vi "ConfigMain_Dash.vi"(10 "ControlsToSave":refnum<vi>[](array[refnum]), 11 "ControlElements":T1) -> ()   [LabVIEW 2015]
uses:
  <vilib>/Rock Robotics/Network Tables/NT Write Boolean.vi
  <vilib>/FTP/NI_FTP.lvlib
panel:
  out "RobotIP":string
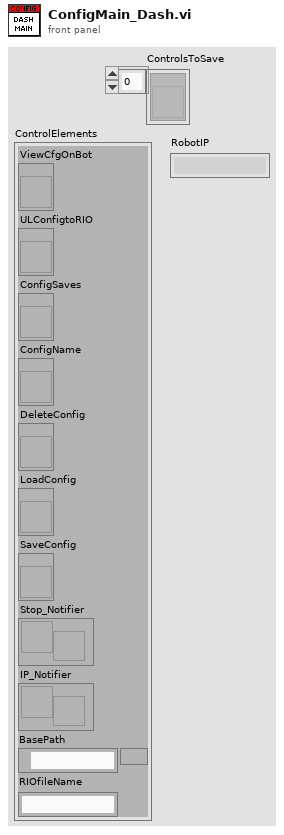
[diagram p1: front panel]
types:
  T1 = cluster{"ViewCfgOnBot":refnum<vi>, "ULConfigtoRIO":refnum<vi>, "ConfigSaves":refnum<vi>, "ConfigName":refnum<vi>, "DeleteConfig":refnum<vi>, "LoadConfig":refnum<vi>, "SaveConfig":refnum<vi>, "Stop_Notifier":refnum<notifier>, "IP_Notifier":refnum<notifier>, "BasePath":path, "RIOfileName":string}
  T2 = enum16{"open", "replace", "create", "open or create", "replace or create", "replace or create with confirmation"}
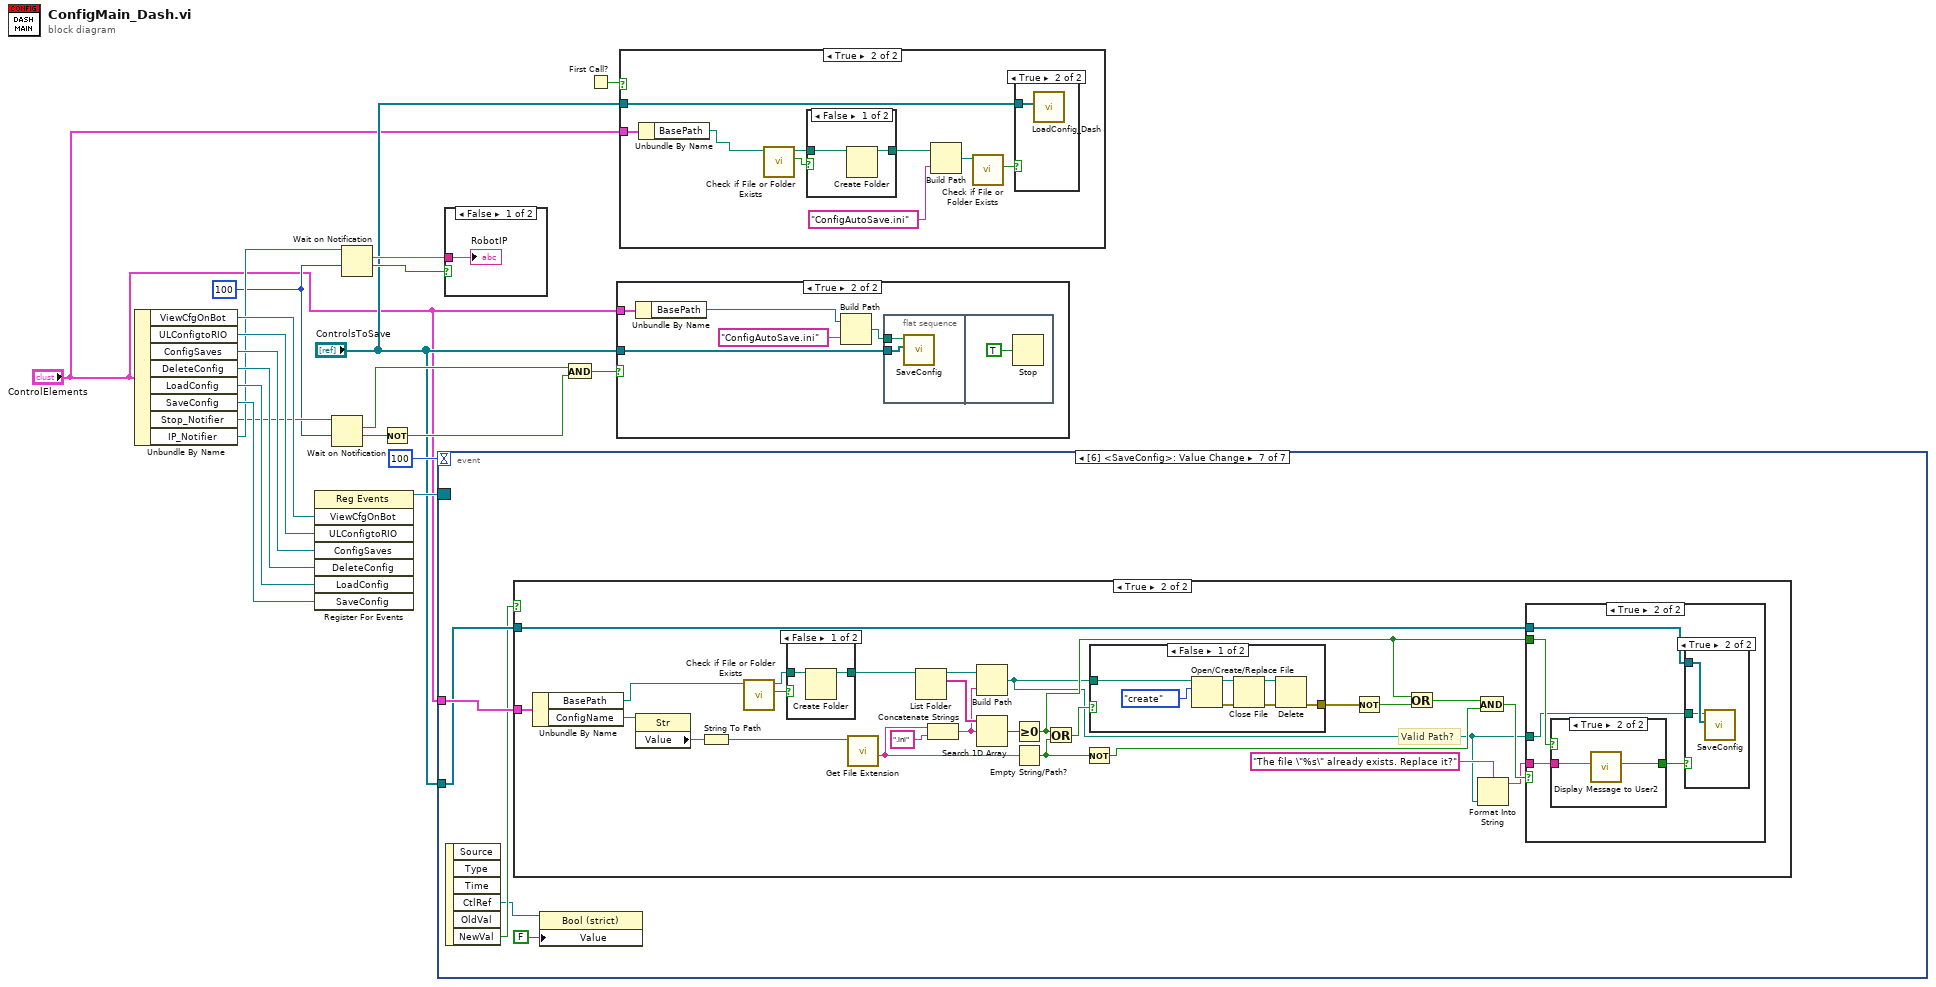
[diagram p0: block diagram]
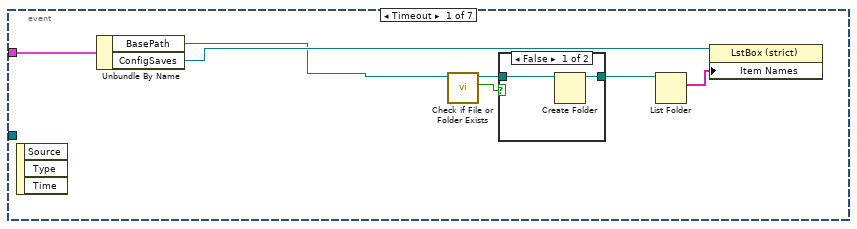
[diagram p7: hidden frame]
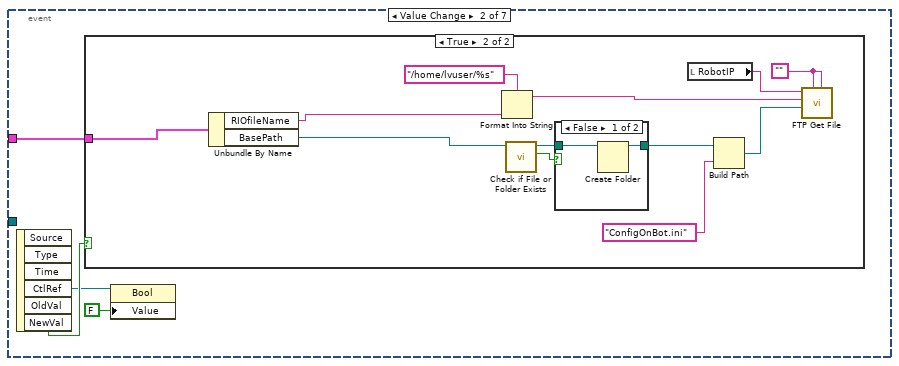
[diagram p9: hidden frame]
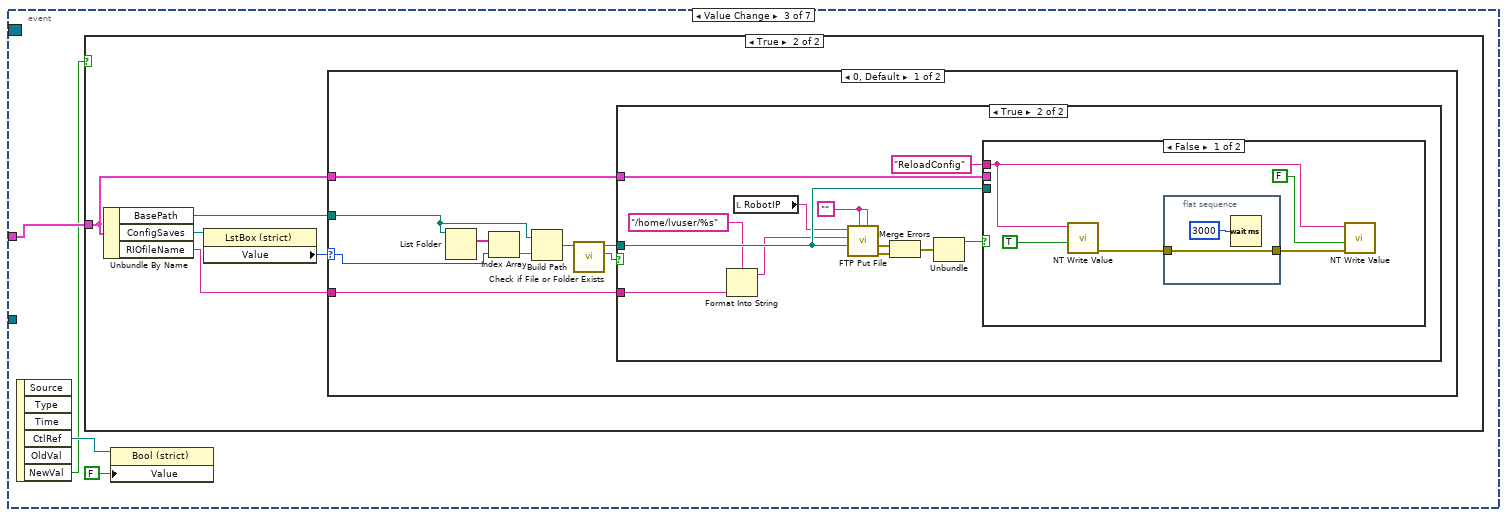
[diagram p12: hidden frame]
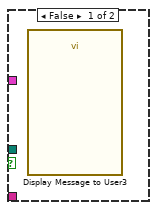
[diagram p14: hidden frame]
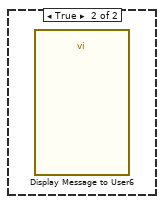
[diagram p15: hidden frame]
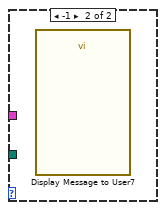
[diagram p16: hidden frame]
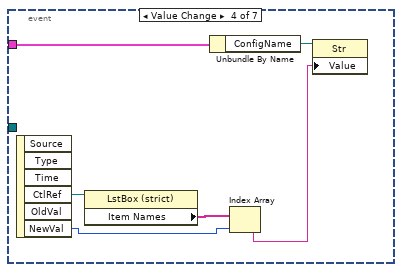
[diagram p17: hidden frame]
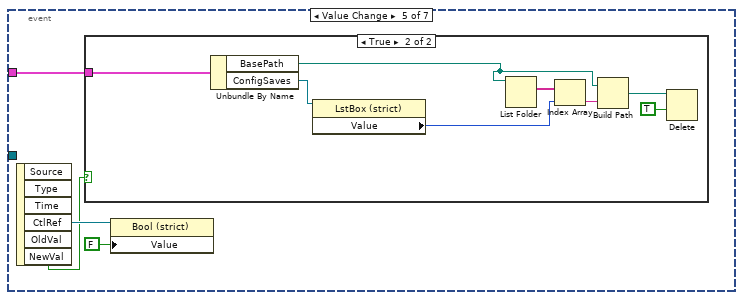
[diagram p18: hidden frame]
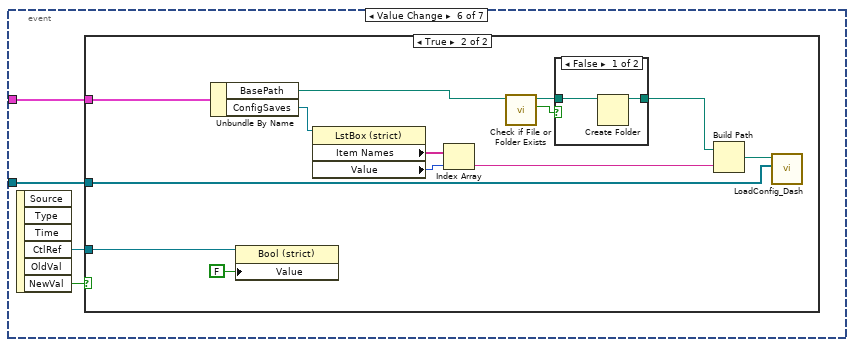
[diagram p20: hidden frame]
diagram:
  w9 = 100 ("timeout in ms (-1)")
  n1 = Unbundle By Name("ControlElements") -> ("ViewCfgOnBot"=w20:refnum<vi>, "ULConfigtoRIO"=w19:refnum<vi>, "ConfigSaves"=w18:refnum<vi>, "DeleteConfig"=w17:refnum<vi>, "LoadConfig"=w16:refnum<vi>, "SaveConfig"=w15:refnum<vi>, "Stop_Notifier"=w13:refnum<notifier>, "IP_Notifier"=w14:refnum<notifier>)
  n2 = register-events(w20, w19, w18, w17, w16, w15) -> (reference out=w12:refnum<event-registration>)  [unwired: 2 in, 1 out]
  n3 = Wait on Notification(notifier=w13, timeout in ms (-1)=w9) -> (notification=w6:bool, timed out?=w8:bool)  [unwired: 2 in, 2 out]
  n4 = Wait on Notification(notifier=w14, timeout in ms (-1)=w9) -> (notification=w11:string, timed out?=w10:bool)  [unwired: 2 in, 2 out]
  n5 = Not(x=w8) -> (.not. x?=w7:bool)
  n6 = event shown="[6] <SaveConfig>: Value Change" {
    selector: w12 -> [_ _ _ _ _ _ _]
    dyn-events: _ -> [_ _ _ _ _ _ _]
    timeout: 100 -> [_ _ _ _ _ _ _]
    tunnel: "ControlElements" -> [w26 w34 w52 w87 w93 w106 w129]
    tunnel: "ControlsToSave" -> [_ _ _ _ _ w105 w128]
    event Timeout {
      n7 = event-data() -> ()  [unwired: 1 in, 3 out]
      n8 = Unbundle By Name(w26) -> ("BasePath"=w21:path, "ConfigSaves"=w27:refnum<vi>)
      n9 = call <vilib>:"Check if File or Folder Exists.vi"("path"=w21) -> ("file or folder exists?"=w24:bool, "dup path"=w23:path)  [unwired: 8 in, 1 out]
      n10 = case shown="False" w24 {
        tunnel: w23 -> [w29 w30]
        tunnel: [w28 w30] -> w22
        frame False {
          n11 = Create Folder(path (use dialog)=w29) -> (created path=w28:path)  [unwired: 2 in, 2 out]
        }
        frame True {
        }
      }
      n12 = List Folder(path=w22) -> (filenames=w25:string[])  [unwired: 3 in, 3 out]
      n13 = property class="LstBox (strict)"(reference=w27, "Item Names"=w25) -> ()  [unwired: 1 in, 2 out]
    }
    event Value Change {
      n14 = event-data() -> ("CtlRef"=w31:refnum<vi>, "NewVal"=w33:bool)  [unwired: 1 in, 4 out]
      n15 = case shown="True" w33 {
        tunnel: w34 -> [_ w40]
        frame False {
        }
        frame True {
          w44 = ""
          n16 = Unbundle By Name(w40) -> ("RIOfileName"=w37:string, "BasePath"=w35:path)
          n17 = Format Into String(format string="/home/lvuser/%s" ("remote path"), w37) -> (resulting string=w36:string)  [unwired: 2 in, 1 out]
          n18 = call <vilib>:"Check if File or Folder Exists.vi"("path"=w35) -> ("file or folder exists?"=w46:bool, "dup path"=w45:path)  [unwired: 8 in, 1 out]
          n19 = case shown="False" w46 {
            tunnel: w45 -> [w48 w49]
            tunnel: [w47 w49] -> w43
            frame False {
              n20 = Create Folder(path (use dialog)=w48) -> (created path=w47:path)  [unwired: 2 in, 2 out]
            }
            frame True {
            }
          }
          n21 = local read "RobotIP"() -> (w39:string)
          n22 = Build Path(base path=w43, name or relative path="ConfigOnBot.ini") -> (appended path=w41:path)
          n23 = call <vilib>:"FTP Get File.vi"("password"=w44, "user"=w44, "local path"=w41, "remote path"=w36, "host"=w39) -> ()  [unwired: 5 in, 2 out]
        }
      }
      n24 = property class="Bool"(reference=w31, "Value"=FALSE ("Panel Transparent")) -> ()  [unwired: 1 in, 2 out]
    }
    event Value Change {
      n25 = event-data() -> ("CtlRef"=w51:refnum<vi>, "NewVal"=w50:bool)  [unwired: 1 in, 4 out]
      n26 = case shown="True" w50 {
        tunnel: w52 -> [_ w56]
        frame False {
        }
        frame True {
          n27 = Unbundle By Name(w56) -> ("BasePath"=w55:path, "ConfigSaves"=w58:refnum<vi>, "RIOfileName"=w54:string)
          n28 = property class="LstBox (strict)"(reference=w58) -> ("Value"=w57:i32)  [unwired: 1 in, 2 out]
          n29 = case shown="0, Default" w57 {
            selector: w57 -> [w65 _]
            tunnel: w56 -> [w61 _]
            tunnel: w55 -> [w60 _]
            tunnel: w54 -> [w59 _]
            frame 0, Default {
              n30 = List Folder(path=w60) -> (filenames=w67:string[])  [unwired: 3 in, 3 out]
              n31 = Index Array(array=w67, index=w65) -> (element=w66:string)
              n32 = Build Path(base path=w60, name or relative path=w66) -> (appended path=w64:path)
              n33 = call <vilib>:"Check if File or Folder Exists.vi"("path"=w64) -> ("file or folder exists?"=w63:bool, "dup path"=w62:path)  [unwired: 8 in, 1 out]
              n34 = case shown="True" w63 {
                tunnel: w62 -> [_ w73]
                tunnel: w61 -> [_ w72]
                tunnel: w59 -> [_ w68]
                frame False {
                  n35 = call "Display Message to User3"() -> ()  [unwired: 10 in, 2 out]
                }
                frame True {
                  w76 = ""
                  n36 = Format Into String(format string="/home/lvuser/%s" ("remote path (roboRIO)"), w68) -> (resulting string=w69:string)  [unwired: 2 in, 1 out]
                  n37 = local read "RobotIP"() -> (w71:string)
                  n38 = call <vilib>:"FTP Put File.vi"("password"=w76, "user"=w76, "local path"=w73, "remote path"=w69, "host"=w71) -> ("error out"=w78:errorcluster, "file error"=w79:errorcluster)  [unwired: 5 in]
                  n39 = Merge Errors(w79, w78) -> (w77:errorcluster)
                  n40 = Unbundle(w77) -> ("status"=w75:bool)  [unwired: 2 out]
                  n41 = case shown="False" w75 {
                    tunnel: "ReloadConfig" ("remote path (roboRIO)") -> [w81 _]
                    tunnel: w73 -> [_ _]
                    tunnel: w72 -> [_ _]
                    frame False {
                      n42 = call-poly <vilib>:"NT Write Value.vi"("Boolean"=TRUE, "Name"=w81) -> ("error out"=w83:errorcluster)  [unwired: 9 in]
                      n43 = flat-sequence {
                        tunnel: w83 -> [w85]
                        tunnel: [w85] -> w82
                        frame #0 {
                          n44 = Wait (ms)(milliseconds to wait=u32 3000) -> ()  [unwired: 1 out]
                        }
                      }
                      n45 = call-poly <vilib>:"NT Write Value.vi"("error in"=w82, "Boolean"=FALSE, "Name"=w81) -> ()  [unwired: 8 in, 1 out]
                    }
                    frame True {
                      n46 = call "Display Message to User6"() -> ()  [unwired: 10 in, 2 out]
                    }
                  }
                }
              }
            }
            frame -1 {
              n47 = call "Display Message to User7"() -> ()  [unwired: 10 in, 2 out]
            }
          }
        }
      }
      n48 = property class="Bool (strict)"(reference=w51, "Value"=FALSE ("Panel Transparent")) -> ()  [unwired: 1 in, 2 out]
    }
    event Value Change {
      n49 = event-data() -> ("CtlRef"=w89:refnum<vi>, "NewVal"=w88:i32)  [unwired: 1 in, 4 out]
      n50 = property class="LstBox (strict)"(reference=w89) -> ("Item Names"=w92:string[])  [unwired: 1 in, 2 out]
      n51 = Unbundle By Name(w87) -> ("ConfigName"=w91:refnum<vi>)
      n52 = Index Array(array=w92, index=w88) -> (element=w90:string)
      n53 = property class="Str"(reference=w91, "Value"=w90) -> ()  [unwired: 1 in, 2 out]
    }
    event Value Change {
      n54 = event-data() -> ("CtlRef"=w95:refnum<vi>, "NewVal"=w94:bool)  [unwired: 1 in, 4 out]
      n55 = case shown="True" w94 {
        tunnel: w93 -> [_ w104]
        frame False {
        }
        frame True {
          n56 = Unbundle By Name(w104) -> ("BasePath"=w97:path, "ConfigSaves"=w103:refnum<vi>)
          n57 = property class="LstBox (strict)"(reference=w103) -> ("Value"=w101:i32)  [unwired: 1 in, 2 out]
          n58 = List Folder(path=w97) -> (filenames=w102:string[])  [unwired: 3 in, 3 out]
          n59 = Index Array(array=w102, index=w101) -> (element=w100:string)
          n60 = Build Path(base path=w97, name or relative path=w100) -> (appended path=w98:path)
          n61 = Delete(path (use dialog)=w98, confirm (F)=TRUE) -> ()  [unwired: 3 in, 3 out]
        }
      }
      n62 = property class="Bool (strict)"(reference=w95, "Value"=FALSE ("Panel Transparent")) -> ()  [unwired: 1 in, 2 out]
    }
    event Value Change {
      n63 = event-data() -> ("CtlRef"=w107:refnum<vi>, "NewVal"=w108:bool)  [unwired: 1 in, 4 out]
      n64 = case shown="True" w108 {
        tunnel: w107 -> [_ w121]
        tunnel: w106 -> [_ w119]
        tunnel: w105 -> [_ w113]
        frame False {
        }
        frame True {
          n65 = Unbundle By Name(w119) -> ("BasePath"=w109:path, "ConfigSaves"=w118:refnum<vi>)
          n66 = property class="Bool (strict)"(reference=w121, "Value"=FALSE) -> ()  [unwired: 1 in, 2 out]
          n67 = property class="LstBox (strict)"(reference=w118) -> ("Item Names"=w116:string[], "Value"=w117:i32)  [unwired: 1 in, 2 out]
          n68 = Index Array(array=w116, index=w117) -> (element=w115:string)
          n69 = call <vilib>:"Check if File or Folder Exists.vi"("path"=w109) -> ("file or folder exists?"=w112:bool, "dup path"=w111:path)  [unwired: 8 in, 1 out]
          n70 = case shown="False" w112 {
            tunnel: w111 -> [w123 w124]
            tunnel: [w122 w124] -> w110
            frame False {
              n71 = Create Folder(path (use dialog)=w123) -> (created path=w122:path)  [unwired: 2 in, 2 out]
            }
            frame True {
            }
          }
          n72 = Build Path(base path=w110, name or relative path=w115) -> (appended path=w114:path)
          n73 = call "LoadConfig_Dash.vi"("ControlsToLoad"=w113, "Path"=w114) -> ()  [unwired: 10 in]
        }
      }
    }
    event Value Change {
      n74 = event-data() -> ("CtlRef"=w125:refnum<vi>, "NewVal"=w127:bool)  [unwired: 1 in, 4 out]
      n75 = case shown="True" w127 {
        tunnel: w129 -> [_ w155]
        tunnel: w128 -> [_ w137]
        frame False {
        }
        frame True {
          # "Valid Path?"
          n76 = Unbundle By Name(w155) -> ("BasePath"=w130:path, "ConfigName"=w154:refnum<vi>)
          n77 = property class="Str"(reference=w154) -> ("Value"=w146:string)  [unwired: 1 in, 2 out]
          n78 = String To Path(string=w146) -> (path=w145:path)
          n79 = call <vilib>:"Check if File or Folder Exists.vi"("path"=w130) -> ("file or folder exists?"=w133:bool, "dup path"=w132:path)  [unwired: 8 in, 1 out]
          n80 = case shown="False" w133 {
            tunnel: w132 -> [w157 w158]
            tunnel: [w156 w158] -> w131
            frame False {
              n81 = Create Folder(path (use dialog)=w157) -> (created path=w156:path)  [unwired: 2 in, 2 out]
            }
            frame True {
            }
          }
          n82 = call <vilib>:"Get File Extension.vi"("file"=w145) -> ("filename without extension"=w144:string)  [unwired: 6 in, 4 out]
          n83 = List Folder(path=w131) -> (path out=w149:path, filenames=w152:string[])  [unwired: 3 in, 2 out]
          n84 = Concatenate Strings(w144, ".ini" ("string")) -> (w147:string)
          n85 = Build Path(base path=w149, name or relative path=w147) -> (appended path=w135:path)
          n86 = Search 1D Array(1D array=w152, element=w147) -> (index of element=w151:i32)  [unwired: 1 in]
          n87 = Greater Or Equal To 0?(x=w151) -> (x >= 0?=w143:bool)
          n88 = Empty String/Path?(string/path=w144) -> (empty?=w140:bool)
          n89 = Or(x=w143, y=w140) -> (x .or. y?=w150:bool)
          n90 = Not(x=w140) -> (.not. x?=w139:bool)
          n91 = case shown="False" w150 {
            tunnel: w135 -> [w175 _]
            tunnel: [w169 _] -> w142
            frame False {
              n92 = Open/Create/Replace File(file path (use dialog)=w175, operation (0:open)=T2."create") -> (refnum out=w172:refnum<file>, error out=w173:errorcluster)  [unwired: 4 in, 1 out]
              n93 = Close File(refnum=w172, error in=w173) -> (path=w170:path, error out=w171:errorcluster)
              n94 = Delete(path (use dialog)=w170, error in=w171) -> (error out=w169:errorcluster)  [unwired: 3 in, 2 out]
            }
            frame True {
            }
          }
          n95 = Not(x=w142) -> (.not. x?=w148:bool)
          n96 = Or(x=w143, y=w148) -> (x .or. y?=w141:bool)
          n97 = And(x=w141, y=w139) -> (x .and. y?=w138:bool)
          n98 = Format Into String(format string="The file \"%s\" already exists. Replace it?", w135) -> (resulting string=w134:string)  [unwired: 2 in, 1 out]
          n99 = case shown="True" w138 {
            tunnel: w143 -> [_ w163]
            tunnel: w137 -> [_ w162]
            tunnel: w135 -> [_ w161]
            tunnel: w134 -> [_ w159]
            frame False {
              n100 = call "Display Message to User"() -> ()  [unwired: 10 in, 2 out]
            }
            frame True {
              n101 = case shown="True" w163 {
                tunnel: [TRUE w167] -> w160
                tunnel: w159 -> [_ w168]
                frame False {
                }
                frame True {
                  n102 = call "Display Message to User2"("Message"=w168) -> ("OK"=w167:bool)  [unwired: 9 in, 1 out]
                }
              }
              n103 = case shown="True" w160 {
                tunnel: w162 -> [_ w165]
                tunnel: w161 -> [_ w164]
                frame False {
                }
                frame True {
                  n104 = call "SaveConfig.vi"("ControlsToSave"=w165, "Path"=w164) -> ()  [unwired: 10 in]
                }
              }
            }
          }
        }
      }
      n105 = property class="Bool (strict)"(reference=w125, "Value"=FALSE) -> ()  [unwired: 1 in, 2 out]
    }
  }
  n106 = case shown="False" w10 {
    tunnel: w11 -> [w176 _]
    frame False {
      "RobotIP" <- w176
    }
    frame True {
    }
  }
  n107 = And(x=w6, y=w7) -> (x .and. y?=w5:bool)
  n108 = First Call?() -> (First Call?: T/F=w1:bool)
  n109 = case shown="True" w5 {
    tunnel: "ControlsToSave" -> [_ w177]
    tunnel: "ControlElements" -> [_ w180]
    frame False {
    }
    frame True {
      n110 = Unbundle By Name(w180) -> ("BasePath"=w179:path)
      n111 = Build Path(base path=w179, name or relative path="ConfigAutoSave.ini") -> (appended path=w178:path)
      n112 = flat-sequence {
        tunnel: w178 -> [w183]
        tunnel: w177 -> [w182]
        frame #0 {
          n113 = call "SaveConfig.vi"("ControlsToSave"=w182, "Path"=w183) -> ()  [unwired: 10 in]
        }
        frame #1 {
          n114 = Stop(stop? (T)=TRUE) -> ()
        }
      }
    }
  }
  n115 = case shown="True" w1 {
    tunnel: "ControlElements" -> [_ w193]
    tunnel: "ControlsToSave" -> [_ w192]
    frame False {
    }
    frame True {
      n116 = Unbundle By Name(w193) -> ("BasePath"=w185:path)
      n117 = call <vilib>:"Check if File or Folder Exists.vi"("path"=w185) -> ("file or folder exists?"=w191:bool, "dup path"=w190:path)  [unwired: 8 in, 1 out]
      n118 = case shown="False" w191 {
        tunnel: w190 -> [w196 w197]
        tunnel: [w195 w197] -> w189
        frame False {
          n119 = Create Folder(path (use dialog)=w196) -> (created path=w195:path)  [unwired: 2 in, 2 out]
        }
        frame True {
        }
      }
      n120 = Build Path(base path=w189, name or relative path="ConfigAutoSave.ini") -> (appended path=w187:path)
      n121 = call <vilib>:"Check if File or Folder Exists.vi"("path"=w187) -> ("file or folder exists?"=w186:bool)  [unwired: 8 in, 2 out]
      n122 = case shown="True" w186 {
        tunnel: w192 -> [_ w194]
        frame False {
        }
        frame True {
          n123 = call "LoadConfig_Dash.vi"("ControlsToLoad"=w194) -> ()  [unwired: 11 in]
        }
      }
    }
  }
